vi "Robot Main.vi"   [LabVIEW 2013]
doc: "This VI imlements the framework and scheduler for your robotics program. It should not be necessary to modify the framework. You are expected to add your code to the VIs called from Robot Main, the ones located in the Team Code within the project."
panel:
  # "2014 Über Test Code"
  # "Version 0.9_Fri: 2-14-14"
  # "PWM"
  # "DIO"
  # "Relay"
  # "Analog"
  # "Solenoid"
  # "1 a): Right Front Drive\n1 b): Right Rear Drive\n2 a): Left Front Drive\n2 b): Left Rear Drive\n3 a): Right Pickup Motor\n3 b): Left Pickup Motor\n     4: Pickup Belt\n     5:  \n     6: \n     7: \n     8: \n     9: \n   10:"
  # "1: Right Drive Encoder A\n  2: Right Drive Encoder B\n  3: Left Drive Encoder A  \n  4: Left Drive Encoder B\n  5: Pickup Motor Encoder A\n  6: Pickup Motor Encoder B\n  7: Shooter Magnetic Sensor R-Up\n  8: Shooter Magnetic Sensor R-Down\n  9: \n10: \n11: \n12: Holding Light Sensor\n13: \n14: Pneumatic Pressure Switch"
  # "1: Compressor Spike\n2:\n3:\n4:\n5:\n6:\n7:\n8:"
  # "1:\n2:\n3:\n4:\n5:\n6:\n7:\n8:"
  # "1: Latch A\n2: Latch B\n3: Shooter A\n4: Shooter B\n5: Shifter A\n6: Shifter B\n7:\n8:"
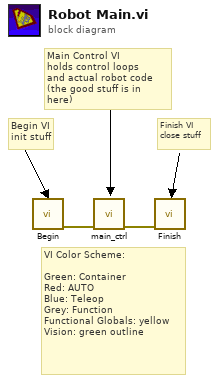
[diagram p0: block diagram]
diagram:
  # "Finish VI\nclose stuff"
  # "Main Control VI\nholds control loops\nand actual robot code\n(the good stuff is in here)"
  # "Begin VI\ninit stuff"
  # "VI Color Scheme:\n\nGreen: Container\nRed: AUTO\nBlue: Teleop\nGrey: Function\nFunctional Globals: yellow\nVision: green outline"
  n1 = call "Begin.vi"() -> ("error out"=w2:errorcluster)  [unwired: 1 in, 10 out]
  n2 = call "main_ctrl.vi"("error in"=w2) -> ("error out"=w1:errorcluster)  [unwired: 10 in]
  n3 = call "Finish.vi"("error in"=w1) -> ()  [unwired: 7 in]
